vi "Logging Message Loop.vi"(8 "error in (no error)":errorcluster, 9 "Data Notifier":refnum<notifier>, 10 "Data Queue":refnum<queue>, 11 "Message Queues":T1) -> (0 "error out":errorcluster)   [LabVIEW 2022 SP3, in "Logging.lvlib"]
doc: "The message loop subVI to handle messages pertaining to logging data."
uses:
  Logging.lvlib
  support/Message Queue/All Message Queues.ctl
  support/Message Queue/Message Cluster.ctl
  QueuedLoggedData.ctl
  FFT-Data.ctl
  Logging Configuration.ctl
  support/TDMS-Refs.ctl
  Logging State.ctl
  FiniteMeasurement-DAQmx/controls/Hardware Configuration.ctl
  AcquisitionFilter.ctl
  support/Message Queue/Enqueue Message (Single).vi
  <vilib>/Utility/error.llb/Error Cluster From Error Code.vi
  <vilib>/ErrorRing/Error Ring.xnode
  support/Message Queue/Message Queue.lvlib
  Acquisition/Acquisition.lvlib
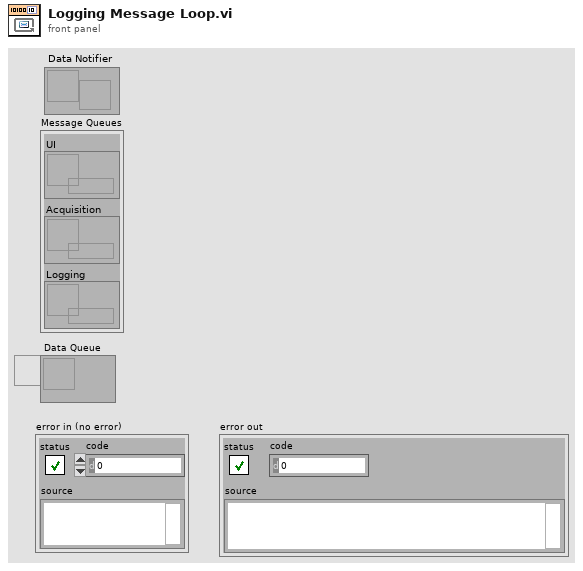
[diagram p1: front panel]
types:
  T1 = typedef "Message Queue.lvlib/All Message Queues.ctl" = cluster{"UI":refnum<queue>, "Acquisition":refnum<queue>, "Logging":refnum<queue>}
  T2 = typedef "Acquisition.lvlib/Hardware Configuration.ctl" = cluster{"Accel-ai0":bool, "Maximum Input":dbl, "Minimum Input":dbl, "Sample Rate":dbl, "Number of Samples":i32, "Accel-ai1":bool, "DAQmx Task":refnum<k21>, "Low Pass Filter":T3}
  T3 = typedef "Acquisition.lvlib/AcquisitionFilter.ctl" = cluster{"Upper Cutoff":dbl, "Lower Cutoff":dbl, "Order":i32}
  T4 = typedef "Logging.lvlib/Logging State.ctl" = cluster{"State":enum16{"Logging", "Not Logging", "Idle"}, "Samples to Save":u32, "Force Trigger":bool, "FFT-Count":i32}
  T5 = typedef "Logging.lvlib/Logging Configuration.ctl" = cluster{"Log File Base Path":path, "Samples to Save":u32, "Acquisition Sample Rate":dbl, "SamplesPerChannel":u32, "FFT - Block Size":u32, "FFT - NumberOfAverages":i32, "Trigger - Time":i32, "Trigger - Threshold":dbl, "Trigger - Channel":u32, "Enable Time Trigger":bool, "Enable Threshold Trigger":bool, "Always Log":bool, "Enable Filter":bool, "FilesRefs":T6, "OutputFileFormat":enum16{"TXT", "TDMS"}, "ActualBlockSize":i32, "HasBeenTriggeredAlready":bool, "Start Time":timestamp}
  T6 = typedef "TDMS-Refs.ctl" = cluster{"TimeDomainTDMSRef":refnum<k34>, "FreuencyDomainTDMSRef":refnum<k34>, "TXT-FileRef":refnum<file>}
  T7 = enum16{"open", "open or create", "create or replace", "create", "open (read-only)"}
  T8 = enum16{"open", "replace", "create", "open or create", "replace or create", "replace or create with confirmation"}
  T9 = typedef "QueuedLoggedData.ctl" = cluster{"RawData":waveform(dbl)[], "FFT ":T10[]}
  T10 = typedef "FFT-Data.ctl" = cluster{"FFT-Mag":cluster{"t0":dbl, "dt":dbl, "Y":dbl[]}, "FFT-Phase":cluster{"t0":dbl, "dt":dbl, "Y":dbl[]}}
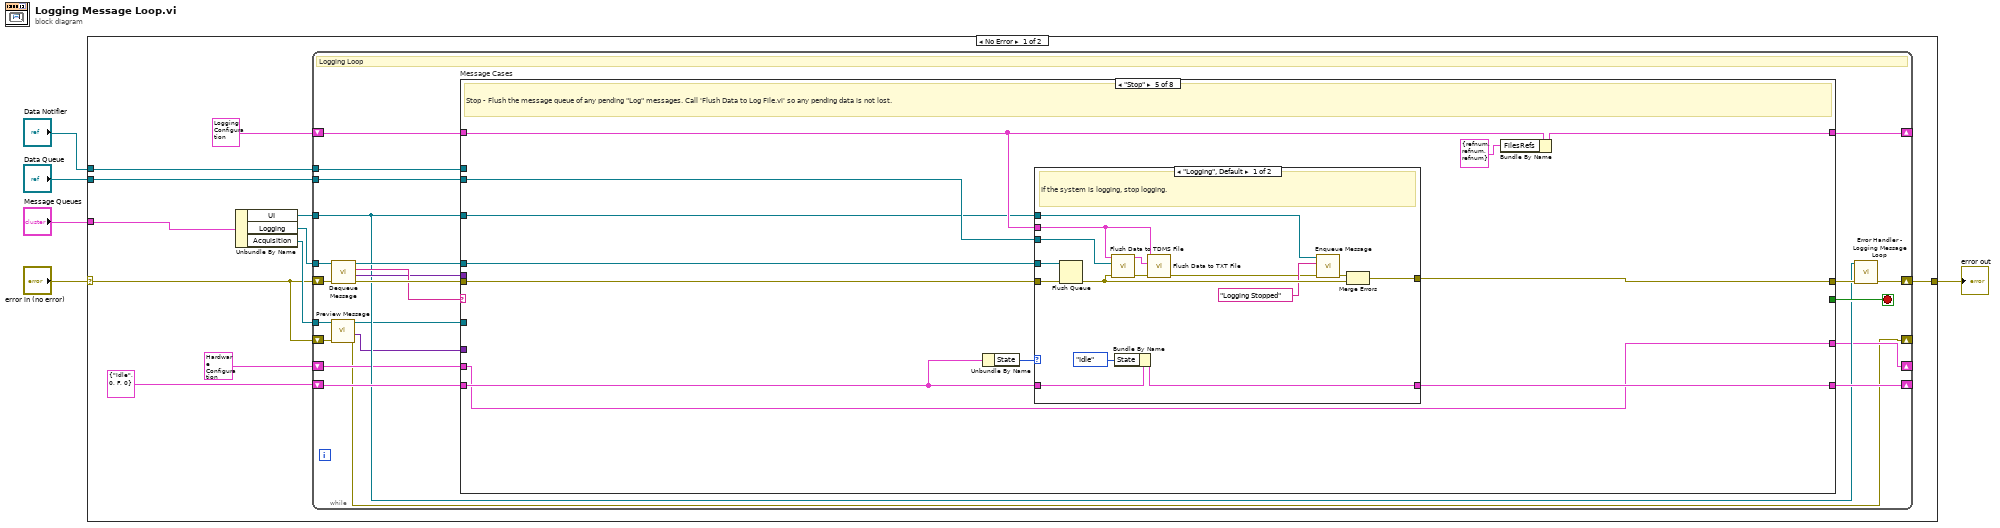
[diagram p0: block diagram]
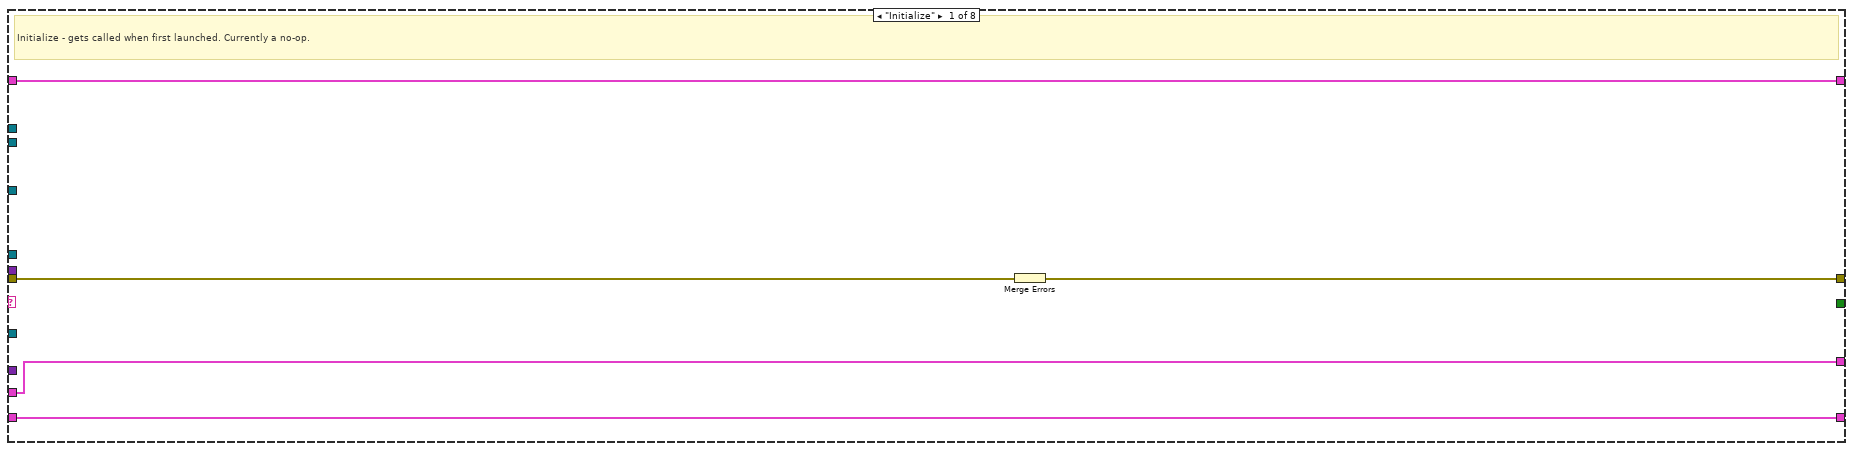
[diagram p2: hidden frame]
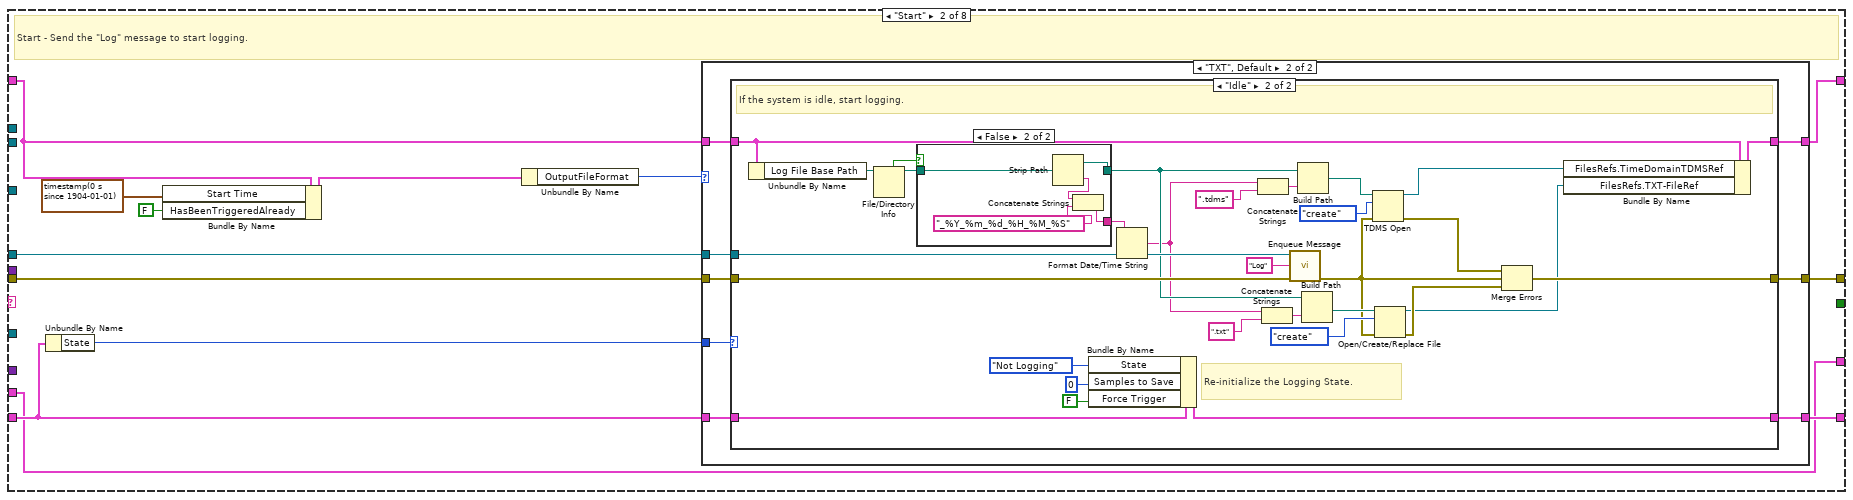
[diagram p3: hidden frame]
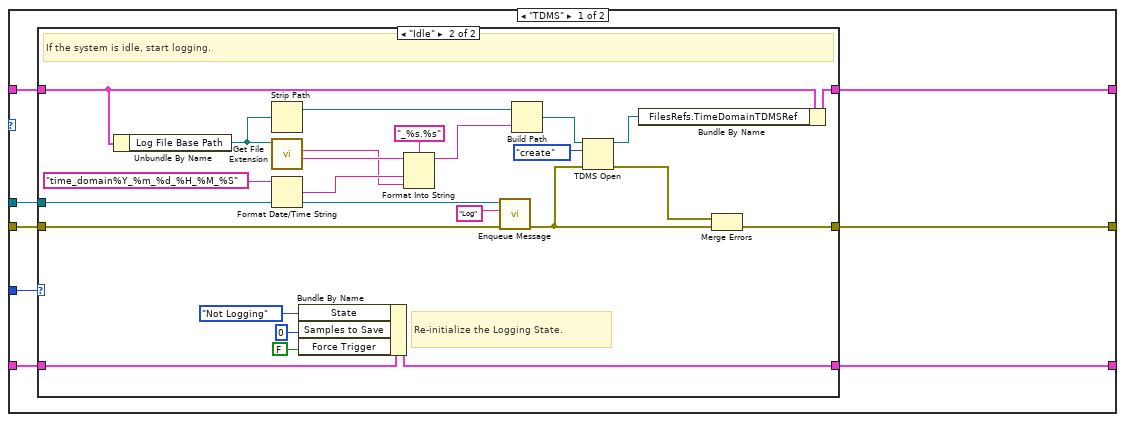
[diagram p4: hidden frame]
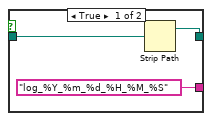
[diagram p7: hidden frame]
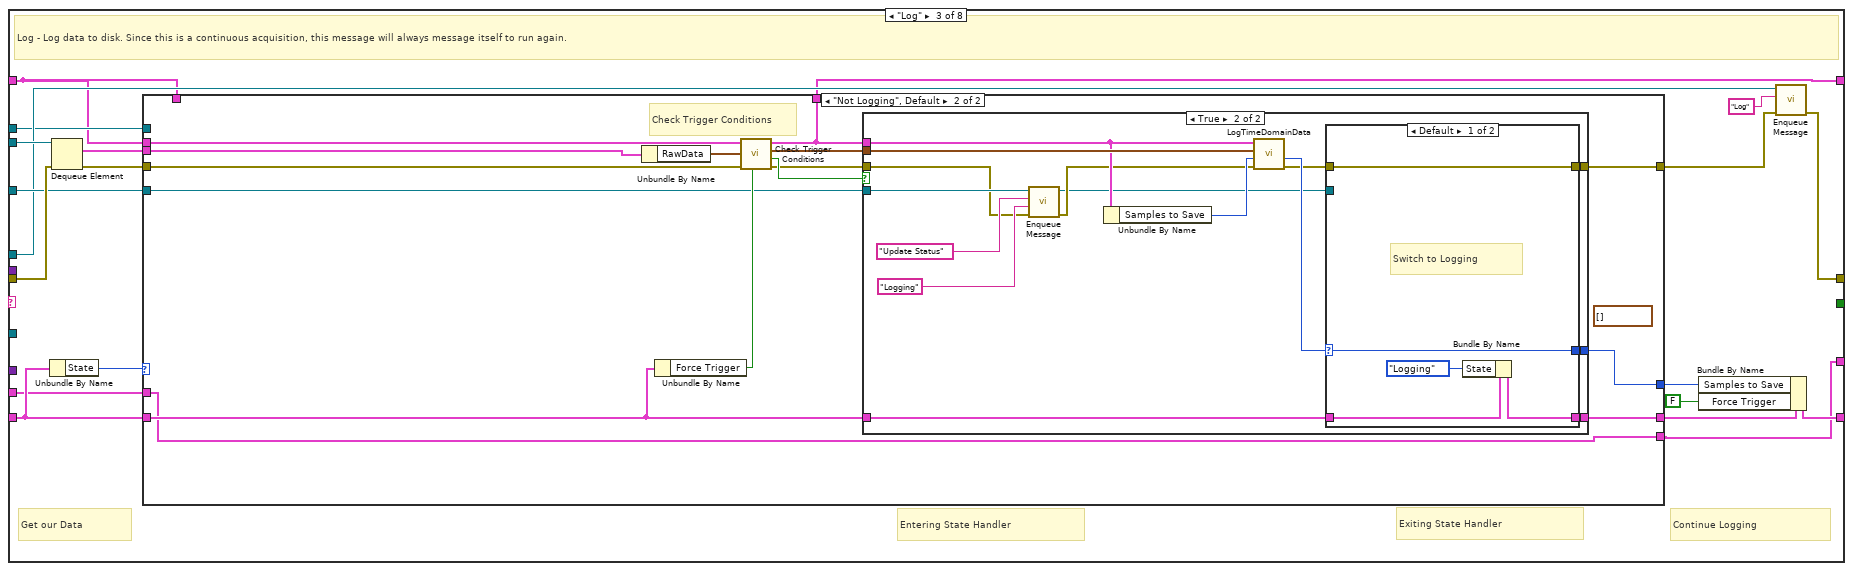
[diagram p8: hidden frame]
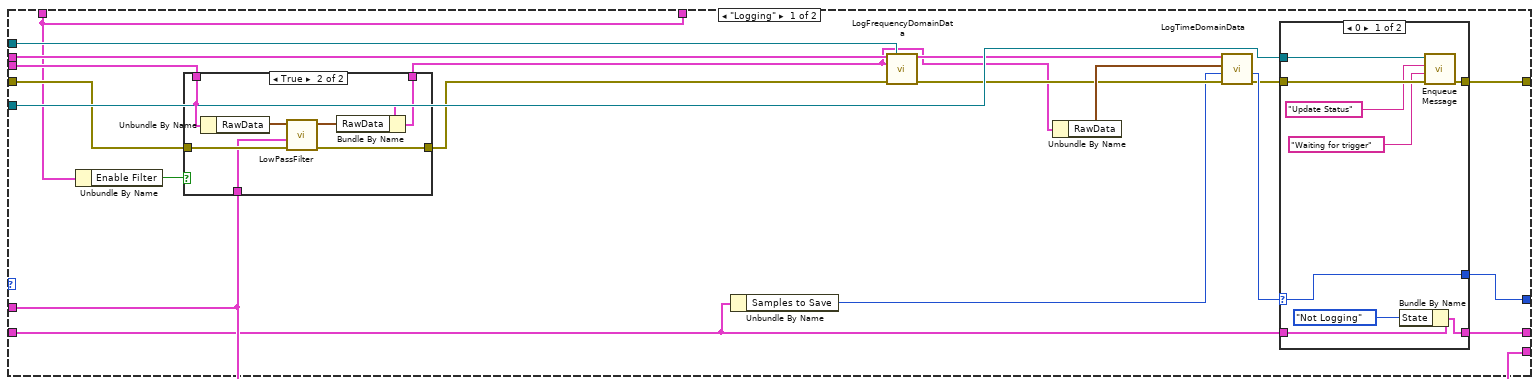
[diagram p9: hidden frame]
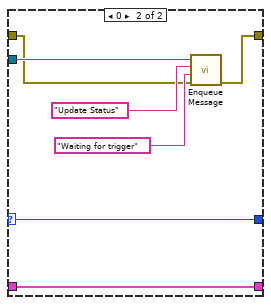
[diagram p13: hidden frame]
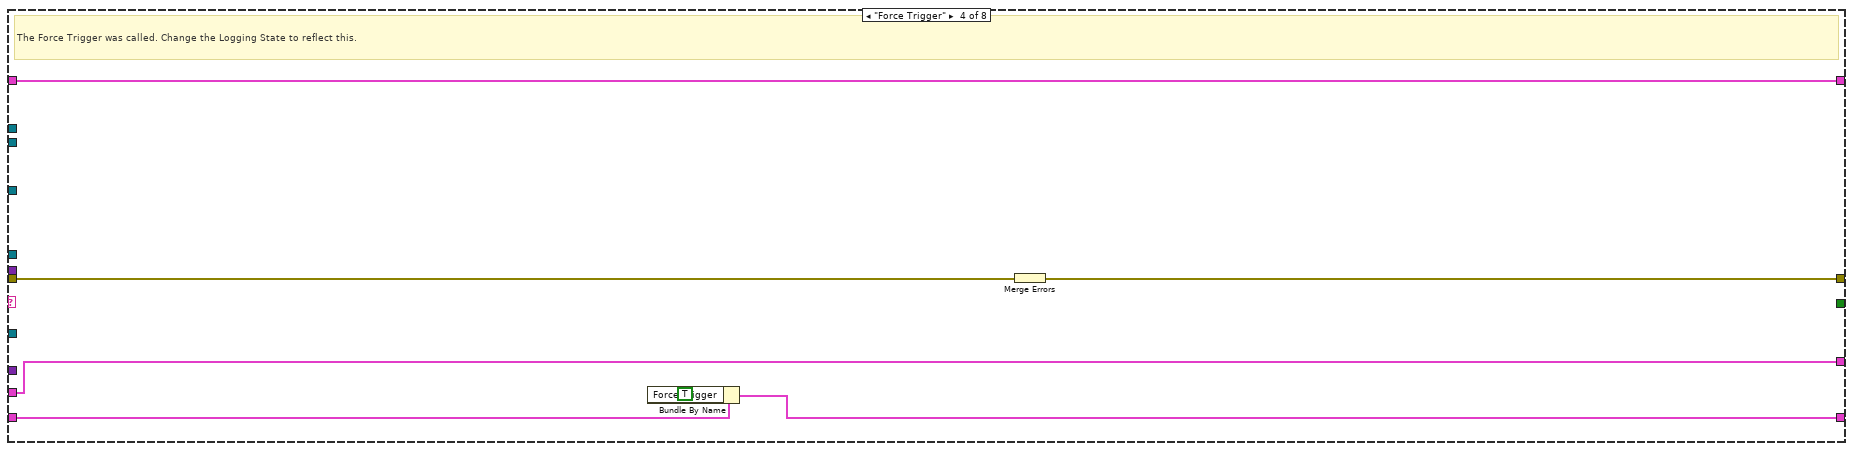
[diagram p14: hidden frame]
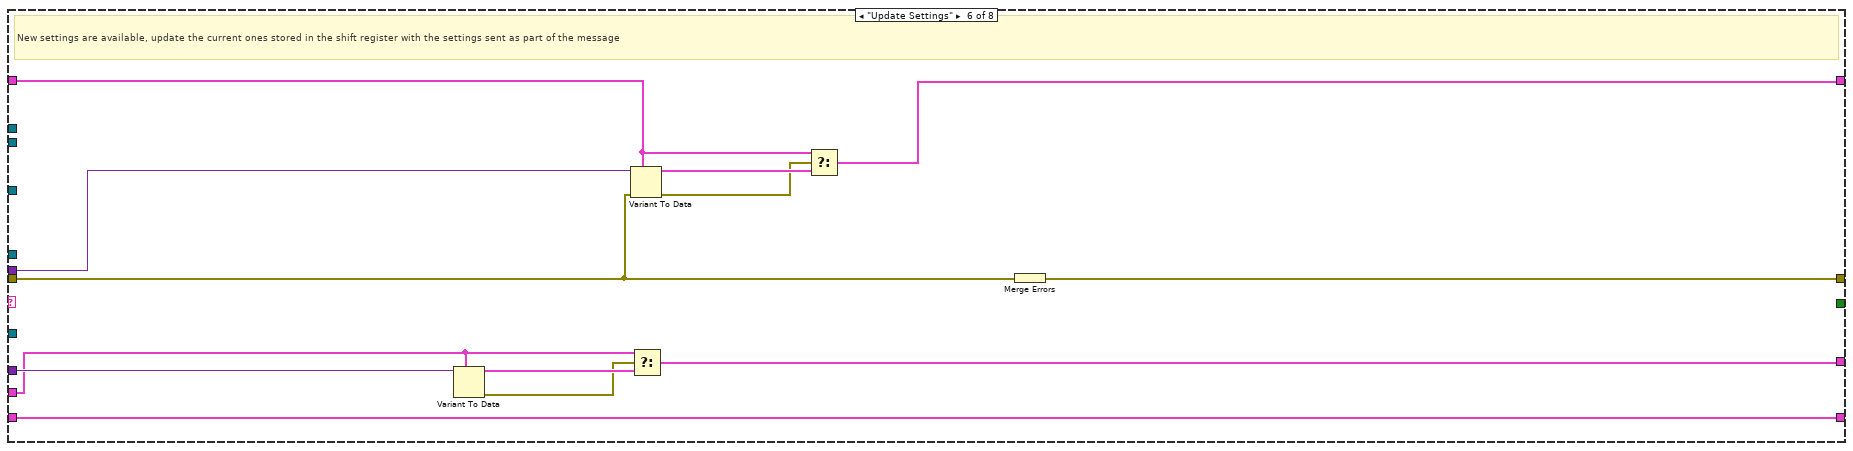
[diagram p16: hidden frame]
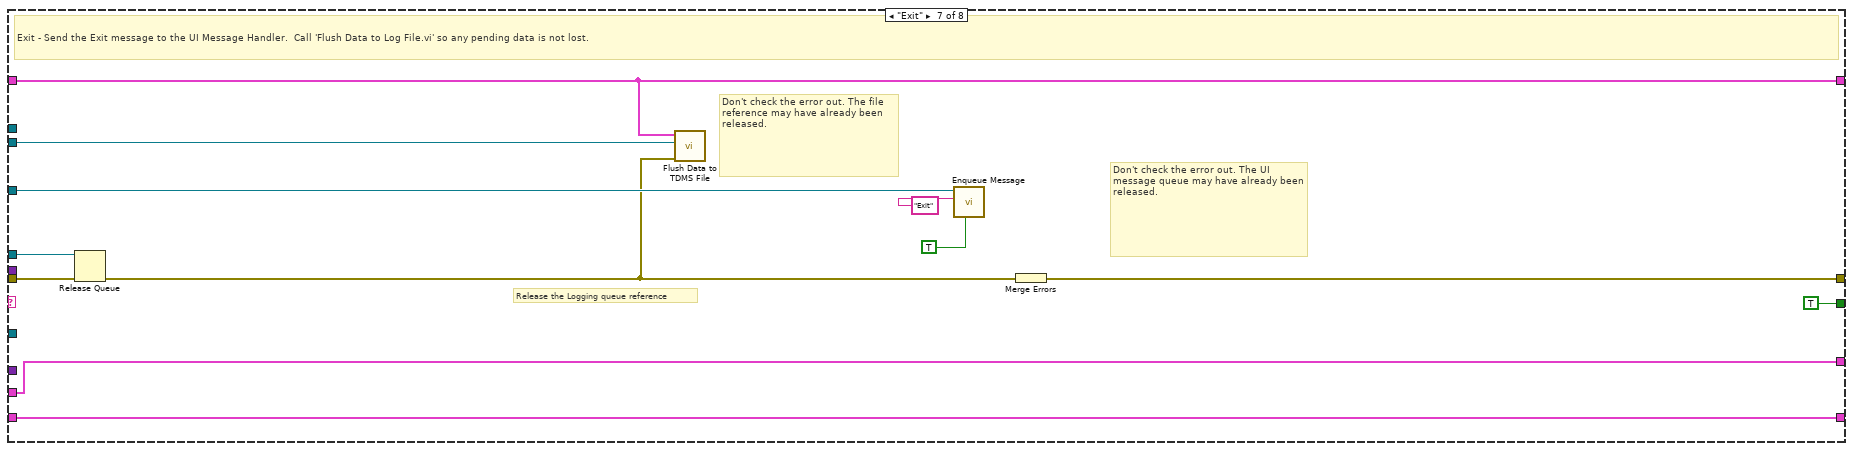
[diagram p17: hidden frame]
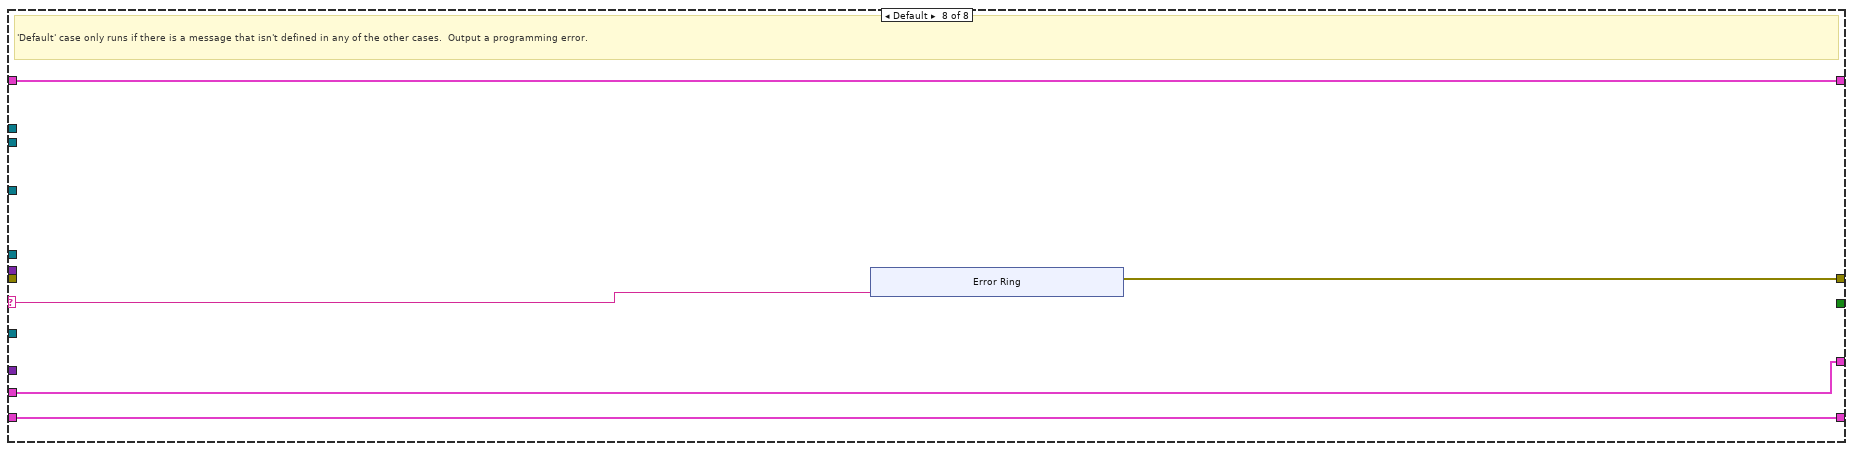
[diagram p18: hidden frame]
diagram:
  n1 = case shown="No Error" "error in (no error)" {
    selector: "error in (no error)" -> [w7 w320]
    tunnel: "Message Queues" -> [w16 _]
    tunnel: [w14 w320] -> w4
    tunnel: "Data Queue" -> [w13 _]
    tunnel: "Data Notifier" -> [w9 _]
    frame No Error {
      n2 = Unbundle By Name(w16) -> ("UI"=w12:refnum<queue>, "Logging"=w15:refnum<queue>, "Acquisition"=w8:refnum<queue>)
      n3 = while {
        tunnel: w15 -> [w31]
        shift-right: [w38] -> _
        shift-left: T5 {"Log File Base Path"=path "", "Samples to Save"=0, "Acquisition Sample Rate"=0.0, "SamplesPerChannel"=0, "FFT - Block Size"=0, "FFT - NumberOfAverages"=0, "Trigger - Time"=0, "Trigger - Threshold"=0.0, "Trigger - Channel"=0, "Enable Time Trigger"=FALSE, "Enable Threshold Trigger"=FALSE, "Always Log"=FALSE, "Enable Filter"=FALSE, "FilesRefs"={"TimeDomainTDMSRef"=refnum, "FreuencyDomainTDMSRef"=refnum, "TXT-FileRef"=refnum}, "OutputFileFormat"=enum."TXT", "ActualBlockSize"=0, "HasBeenTriggeredAlready"=FALSE, "Start Time"=timestamp(0 s since 1904-01-01)} ("Logging Configuration") -> [w39]
        shift-right: [w26] -> w14
        shift-left: w7 -> [w36]
        tunnel: w12 -> [w25]
        tunnel: w13 -> [w30]
        shift-right: [w28] -> _
        shift-left: T4 {"State"=enum."Idle", "Samples to Save"=0, "Force Trigger"=FALSE, "FFT-Count"=0} -> [w29]
        tunnel: w9 -> [w24]
        tunnel: w8 -> [w23]
        shift-right: [w17] -> _
        shift-left: w7 -> [w22]
        shift-right: [w18] -> _
        shift-left: T2 {"Accel-ai0"=FALSE, "Maximum Input"=0.0, "Minimum Input"=0.0, "Sample Rate"=0.0, "Number of Samples"=0, "Accel-ai1"=FALSE, "DAQmx Task"="", "Low Pass Filter"={"Upper Cutoff"=350.0, "Lower Cutoff"=350.0, "Order"=350}} ("Hardware Configuration") -> [w20]
        stop <- w37 stop-if-true
        # "Logging Loop"
        n4 = call "Preview Message.vi"("error in (no error)"=w22, "Message Queue"=w23) -> ("error out"=w17:errorcluster, "Message Data"=w19:variant, "dup Message Queue"=w21:refnum<queue>)  [unwired: 6 in, 1 out]
        n5 = call "Dequeue Message.vi"("error in (no error)"=w36, "Message Queue"=w31) -> ("error out"=w35:errorcluster, "Message Data"=w33:variant, "Message"=w34:string, "dup Message Queue"=w32:refnum<queue>)  [unwired: 6 in]
        n6 = case "Message Cases" shown="\"Stop\"" w34 {
          selector: w34 -> [_ _ _ _ _ _ _ w309]
          tunnel: w32 -> [_ w56 w151 _ w263 _ w301 _]
          tunnel: w35 -> [w42 w55 w160 w253 w264 w289 w304 _]
          tunnel: [w44 w57 w161 w251 w265 w295 w306 w310] -> w27
          tunnel: w39 -> [w43 w50 w142 w252 w261 w293 w300 w312]
          tunnel: [w43 w54 w143 w252 w262 w290 w300 w312] -> w38
          tunnel: [_ _ _ _ _ _ TRUE _] -> w37
          tunnel: w33 -> [_ _ _ _ _ w294 _ _]
          tunnel: w25 -> [_ _ w155 _ w259 _ w305 _]
          tunnel: w30 -> [_ _ w152 _ w260 _ w299 _]
          tunnel: w29 -> [w41 w52 w158 w250 w257 w288 w297 w311]
          tunnel: [w41 w53 w154 w249 w256 w288 w297 w311] -> w28
          tunnel: w24 -> [_ _ w146 _ _ _ _ _]
          tunnel: w21 -> [_ _ _ _ _ _ _ _]
          tunnel: w20 -> [w40 w48 w145 w247 w254 w284 w296 w308]
          tunnel: w19 -> [_ _ _ _ _ w285 _ _]
          tunnel: [w40 w48 w144 w247 w254 w283 w296 w308] -> w18
          frame "Initialize" {
            # "Initialize - gets called when first launched. Currently a no-op."
            n7 = Merge Errors(w42) -> (w44:errorcluster)
          }
          frame "Start" {
            # "Start - Send the \"Log\" message to start logging."
            n8 = Unbundle By Name(w52) -> ("State"=w51:enum16{"Logging", "Not Logging", "Idle"})
            n9 = Bundle By Name(cluster=w50, "Start Time"=timestamp(0 s since 1904-01-01), "HasBeenTriggeredAlready"=FALSE) -> (w47:T5)
            n10 = Unbundle By Name(w47) -> ("OutputFileFormat"=w49:enum16{"TXT", "TDMS"})
            n11 = case shown="\"TXT\", Default" w49 {
              tunnel: [w65 w100] -> w57
              tunnel: w56 -> [w64 w99]
              tunnel: w55 -> [w63 w98]
              tunnel: [w62 w97] -> w54
              tunnel: [w61 w96] -> w53
              tunnel: w52 -> [w60 w95]
              tunnel: w51 -> [w59 w94]
              tunnel: w50 -> [w58 w93]
              frame "TDMS" {
                n12 = case shown="\"Idle\"" w59 {
                  tunnel: [w67 w92] -> w65
                  tunnel: w64 -> [_ w91]
                  tunnel: w63 -> [w67 w89]
                  tunnel: w58 -> [w68 w80]
                  tunnel: [w68 w77] -> w62
                  tunnel: w60 -> [w66 w73]
                  tunnel: [w66 w72] -> w61
                  frame "Logging", Default {
                    # "The system is already running. Ignore the \"Start\" message."
                  }
                  frame "Idle" {
                    # "Re-initialize the Logging State."
                    # "If the system is idle, start logging."
                    n13 = Unbundle By Name(w80) -> ("Log File Base Path"=w87:path)
                    n14 = Strip Path(path=w87) -> (stripped path=w86:path)  [unwired: 1 out]
                    n15 = call <vilib>:"Get File Extension.vi"("file"=w87) -> ("filename without extension"=w85:string, "lowercase file extension"=w82:string)  [unwired: 6 in, 3 out]
                    n16 = Format Date/Time String(time format string (%c)="time_domain%Y_%m_%d_%H_%M_%S") -> (date/time string=w83:string)  [unwired: 2 in]
                    n17 = Bundle By Name(cluster=w73, "State"=enum16{"Logging", "Not Logging"}."Not Logging", "Samples to Save"=u32 0 ("Reads to Save"), "Force Trigger"=FALSE) -> (w72:T4)
                    n18 = Format Into String(format string="_%s.%s", initial string=w85, w83, w82) -> (resulting string=w81:string)  [unwired: 1 in, 1 out]
                    n19 = call-poly "Enqueue Message.vi"("error in (no error)"=w89, "Message"="Log", "Message Queue"=w91) -> ("error out"=w75:errorcluster)  [unwired: 7 in, 1 out]
                    n20 = Build Path(base path=w86, name or relative path=w81) -> (appended path=w78:path)
                    n21 = TDMS Open(8:w75, 10:T7."create" ("operation (0:open)"), 11:w78) -> (0:w74:errorcluster, 3:w79:refnum<k34>)  [unwired: 4 in]
                    n22 = Bundle By Name(cluster=w80, "FilesRefs.TimeDomainTDMSRef"=w79) -> (w77:T5)
                    n23 = Merge Errors(w74, w75) -> (w92:errorcluster)
                  }
                }
              }
              frame "TXT", Default {
                n24 = case shown="\"Idle\"" w94 {
                  tunnel: [w102 w133] -> w100
                  tunnel: w99 -> [_ w132]
                  tunnel: w98 -> [w102 w130]
                  tunnel: w93 -> [w103 w128]
                  tunnel: [w103 w125] -> w97
                  tunnel: w95 -> [w101 w122]
                  tunnel: [w101 w121] -> w96
                  frame "Logging", Default {
                    # "The system is already running. Ignore the \"Start\" message."
                  }
                  frame "Idle" {
                    # "Re-initialize the Logging State."
                    # "If the system is idle, start logging."
                    n25 = Unbundle By Name(w128) -> ("Log File Base Path"=w117:path)
                    n26 = File/Directory Info(path=w117) -> (path out=w105:path, directory=w104:bool)  [unwired: 1 in, 5 out]
                    n27 = case shown="False" w104 {
                      tunnel: ["log_%Y_%m_%d_%H_%M_%S" ("time format string (%c)") w137] -> w129
                      tunnel: [w135 w141] -> w107
                      tunnel: w105 -> [w134 w140]
                      frame True {
                        n28 = Strip Path(path=w134) -> (stripped path=w135:path)  [unwired: 1 out]
                      }
                      frame False {
                        n29 = Strip Path(path=w140) -> (stripped path=w141:path, name=w139:string)
                        n30 = Concatenate Strings(w139, "_%Y_%m_%d_%H_%M_%S" ("time format string (%c)")) -> (w137:string)
                      }
                    }
                    n31 = Bundle By Name(cluster=w122, "State"=enum16{"Logging", "Not Logging"}."Not Logging", "Samples to Save"=u32 0 ("Reads to Save"), "Force Trigger"=FALSE) -> (w121:T4)
                    n32 = Format Date/Time String(time format string (%c)=w129) -> (date/time string=w106:string)  [unwired: 2 in]
                    n33 = Concatenate Strings(w106, ".tdms" ("input 2")) -> (w116:string)
                    n34 = Concatenate Strings(w106, ".txt" ("input 2")) -> (w114:string)
                    n35 = call-poly "Enqueue Message.vi"("error in (no error)"=w130, "Message"="Log", "Message Queue"=w132) -> ("error out"=w110:errorcluster)  [unwired: 7 in, 1 out]
                    n36 = Build Path(base path=w107, name or relative path=w116) -> (appended path=w126:path)
                    n37 = Build Path(base path=w107, name or relative path=w114) -> (appended path=w112:path)
                    n38 = TDMS Open(8:w110, 10:T7."create" ("operation (0:open)"), 11:w126) -> (0:w123:errorcluster, 3:w127:refnum<k34>)  [unwired: 4 in]
                    n39 = Open/Create/Replace File(file path (use dialog)=w112, error in=w110, operation (0:open)=T8."create") -> (refnum out=w108:refnum<file>, error out=w109:errorcluster)  [unwired: 3 in, 1 out]
                    n40 = Merge Errors(w123, w110, w109) -> (w133:errorcluster)
                    n41 = Bundle By Name(cluster=w128, "FilesRefs.TimeDomainTDMSRef"=w127, "FilesRefs.TXT-FileRef"=w108) -> (w125:T5)
                  }
                }
              }
            }
          }
          frame "Log" {
            # "Exiting State Handler"
            # "Continue Logging"
            # "Entering State Handler"
            # "Get our Data"
            # "Log - Log data to disk. Since this is a continuous acquisition, this message will always message itself to run again."
            n42 = Unbundle By Name(w158) -> ("State"=w159:enum16{"Logging", "Not Logging", "Idle"})
            n43 = Dequeue Element(queue=w152, error in (no error)=w160) -> (element=w157:T9, error out=w156:errorcluster)  [unwired: 1 in, 2 out]
            n44 = case shown="\"Not Logging\", Default" w159 {
              tunnel: [w180 w210] -> w150
              tunnel: w158 -> [w163 w208]
              tunnel: w157 -> [w166 w216]
              tunnel: w156 -> [w169 w215]
              tunnel: w142 -> [w172 w217]
              tunnel: w155 -> [w176 w207]
              tunnel: [w177 w209] -> w149
              tunnel: [w179 w206] -> w148
              tunnel: w146 -> [w170 _]
              tunnel: w142 -> [w162 _]
              tunnel: w145 -> [w164 w204]
              tunnel: [w164 w204] -> w144
              tunnel: [w162 w203] -> w143
              frame "Logging" {
                n45 = Unbundle By Name(w162) -> ("Enable Filter"=w165:bool)
                n46 = case shown="True" w165 {
                  tunnel: w169 -> [w183 w189]
                  tunnel: [w183 w188] -> w168
                  tunnel: [w182 w186] -> w167
                  tunnel: w166 -> [w182 w185]
                  tunnel: w164 -> [_ w184]
                  frame False {
                  }
                  frame True {
                    n47 = Unbundle By Name(w185) -> ("RawData"=w190:waveform(dbl)[])
                    n48 = call "LowPassFilter.vi"("error in (no error)"=w189, "Àcquiring Configurations"=w184, "InputData"=w190) -> ("error out"=w188:errorcluster, "OutputData"=w187:waveform(dbl)[])  [unwired: 7 in]
                    n49 = Bundle By Name(cluster=w185, "RawData"=w187) -> (w186:T9)
                  }
                }
                n50 = Unbundle By Name(w163) -> ("Samples to Save"=w171:u32)
                n51 = call "LogFrequencyDomainData.vi"("Logging Configuration Input"=w172, "Data Notifier"=w170, "QueuedDataInput"=w167, "error in (no error)"=w168) -> ("Logging Configuration Output"=w173:T5, "error out"=w174:errorcluster)  [unwired: 10 in]
                n52 = Unbundle By Name(w167) -> ("RawData"=w175:waveform(dbl)[])
                n53 = call "LogTimeDomainData.vi"("error in (no error)"=w174, "Samples to Save In"=w171, "Data"=w175, "Logging Configuration"=w173) -> ("error out"=w178:errorcluster, "Samples to Save Out"=w181:u32)  [unwired: 6 in]
                n54 = case shown="0" w181 {
                  selector: w181 -> [w196 w202]
                  tunnel: w178 -> [w194 w201]
                  tunnel: [w195 w201] -> w177
                  tunnel: w163 -> [w198 w200]
                  tunnel: [w197 w200] -> w180
                  tunnel: [w196 w202] -> w179
                  tunnel: w176 -> [w191 _]
                  frame 0 {
                    n55 = Bundle By Name(cluster=w198, "State"=enum16{"Logging", "Not Logging"}."Not Logging") -> (w197:T4)
                    n56 = call-poly "Enqueue Message.vi"("error in (no error)"=w194, "Message Data"="Waiting for trigger" ("Waiting for trigger"), "Message"="Update Status", "Message Queue"=w191) -> ("error out"=w195:errorcluster)  [unwired: 6 in, 1 out]
                  }
                  frame Default {
                    # "Continue in our same State."
                  }
                }
              }
              frame "Not Logging", Default {
                (unwired) waveform(dbl)[] []
                # "Check Trigger Conditions"
                n57 = Unbundle By Name(w216) -> ("RawData"=w205:waveform(dbl)[])
                n58 = Unbundle By Name(w208) -> ("Force Trigger"=w214:bool)
                n59 = call "Check Trigger Conditions.vi"("Force Trigger?"=w214, "error in (no error)"=w215, "Waveform Data In"=w205, "Logging Configuration In"=w217) -> ("error out"=w212:errorcluster, "Trigger Conditions Met?"=w213:bool, "Waveform Data Out (copy)"=w211:waveform(dbl)[], "Logging Configuration Out"=w203:T5)  [unwired: 4 in]
                n60 = case shown="True" w213 {
                  tunnel: w212 -> [w218 w228]
                  tunnel: w211 -> [_ w234]
                  tunnel: w203 -> [_ w233]
                  tunnel: w208 -> [w219 w224]
                  tunnel: [w219 w223] -> w210
                  tunnel: [w218 w221] -> w209
                  tunnel: w207 -> [_ w232]
                  tunnel: [_ w225] -> w206
                  frame False {
                  }
                  frame True {
                    n61 = call-poly "Enqueue Message.vi"("error in (no error)"=w228, "Message Data"="Logging" ("Logging"), "Message"="Update Status", "Message Queue"=w232) -> ("error out"=w227:errorcluster, "dup Message Queue"=w220:refnum<queue>)  [unwired: 6 in]
                    n62 = Unbundle By Name(w233) -> ("Samples to Save"=w229:u32)
                    n63 = call "LogTimeDomainData.vi"("error in (no error)"=w227, "Samples to Save In"=w229, "Data"=w234, "Logging Configuration"=w233) -> ("error out"=w222:errorcluster, "Samples to Save Out"=w226:u32)  [unwired: 6 in]
                    n64 = case shown="Default" w226 {
                      selector: w226 -> [w239 w246]
                      tunnel: [w239 w246] -> w225
                      tunnel: [w236 w245] -> w223
                      tunnel: w224 -> [w237 w245]
                      tunnel: w222 -> [w235 w241]
                      tunnel: [w235 w240] -> w221
                      tunnel: w220 -> [_ w244]
                      frame Default {
                        # "Switch to Logging"
                        n65 = Bundle By Name(cluster=w237, "State"=enum16{"Logging", "Not Logging"}."Logging") -> (w236:T4)
                      }
                      frame 0 {
                        n66 = call-poly "Enqueue Message.vi"("error in (no error)"=w241, "Message Data"="Waiting for trigger" ("Waiting for trigger"), "Message"="Update Status", "Message Queue"=w244) -> ("error out"=w240:errorcluster)  [unwired: 6 in, 1 out]
                      }
                    }
                  }
                }
              }
            }
            n67 = Bundle By Name(cluster=w150, "Samples to Save"=w148, "Force Trigger"=FALSE) -> (w154:T4)
            n68 = call-poly "Enqueue Message.vi"("error in (no error)"=w149, "Message"="Log", "Message Queue"=w151) -> ("error out"=w161:errorcluster)  [unwired: 7 in, 1 out]
          }
          frame "Force Trigger" {
            # "The Force Trigger was called. Change the Logging State to reflect this."
            n69 = Bundle By Name(cluster=w250, "Force Trigger"=TRUE) -> (w249:T4)
            n70 = Merge Errors(w253) -> (w251:errorcluster)
          }
          frame "Stop" {
            # "Stop - Flush the message queue of any pending \"Log\" messages. Call 'Flush Data to Log File.vi' so any pending data is not lost."
            n71 = Unbundle By Name(w257) -> ("State"=w258:enum16{"Logging", "Not Logging", "Idle"})
            n72 = case shown="\"Logging\", Default" w258 {
              tunnel: [w280 w282] -> w265
              tunnel: w264 -> [w279 w282]
              tunnel: w263 -> [w278 _]
              tunnel: w261 -> [w266 _]
              tunnel: w260 -> [w277 _]
              tunnel: w259 -> [w273 _]
              tunnel: w257 -> [w271 w281]
              tunnel: [w270 w281] -> w256
              frame "Logging", Default {
                # "If the system is logging, stop logging."
                n73 = Flush Queue(queue=w278, error in (no error)=w279) -> (error out=w276:errorcluster)  [unwired: 2 out]
                n74 = call "Flush Data to TDMS File.vi"("error in (no error)"=w276, "Data Queue"=w277, "Logging Configuration"=w266) -> ("error out"=w275:errorcluster, "remaining elements"=w267:T9[])  [unwired: 7 in]
                n75 = Bundle By Name(cluster=w271, "State"=enum16{"Logging", "Not Logging", "Idle"}."Idle") -> (w270:T4)
                n76 = call "Flush Data to TXT File.vi"("error in (no error)"=w275, "remaining elements"=w267, "Logging Configuration Input"=w266) -> ("error out"=w268:errorcluster)  [unwired: 8 in]
                n77 = call-poly "Enqueue Message.vi"("error in (no error)"=w268, "Message"="Logging Stopped", "Message Queue"=w273) -> ("error out"=w274:errorcluster)  [unwired: 7 in, 1 out]
                n78 = Merge Errors(w274, w276) -> (w280:errorcluster)
              }
              frame "Idle" {
                # "The system is already idle. Ignore the \"Stop\" message."
              }
            }
            n79 = Bundle By Name(cluster=w261, "FilesRefs"=T6 {"TimeDomainTDMSRef"=refnum, "FreuencyDomainTDMSRef"=refnum, "TXT-FileRef"=refnum}) -> (w262:T5)
          }
          frame "Update Settings" {
            # "New settings are available, update the current ones stored in the shift register with the settings sent as part of the message"
            n80 = Variant To Data(type=w284, Variant=w285) -> (data=w287:T2, error out=w286:errorcluster)  [unwired: 1 in]
            n81 = Variant To Data(error in=w289, type=w293, Variant=w294) -> (data=w292:T5, error out=w291:errorcluster)
            n82 = Select(t=w284, s=w286, f=w287) -> (s? t:f=w283:T2)
            n83 = Select(t=w293, s=w291, f=w292) -> (s? t:f=w290:T5)
            n84 = Merge Errors(w289) -> (w295:errorcluster)
          }
          frame "Exit" {
            # "Don't check the error out. The file reference may have already been released."
            # "Release the Logging queue reference"
            # "Don't check the error out. The UI message queue may have already been released."
            # "Exit - Send the Exit message to the UI Message Handler.  Call 'Flush Data to Log File.vi' so any pending data is not lost."
            n85 = Release Queue(queue=w301, error in (no error)=w304) -> (error out=w298:errorcluster)  [unwired: 1 in, 2 out]
            n86 = call "Flush Data to TDMS File.vi"("error in (no error)"=w298, "Data Queue"=w299, "Logging Configuration"=w300) -> ()  [unwired: 7 in, 2 out]
            n87 = call-poly "Enqueue Message.vi"("Priority Message? (F)"=TRUE, "Message"="Exit", "Message Queue"=w305) -> ()  [unwired: 7 in, 2 out]
            n88 = Merge Errors(w298) -> (w306:errorcluster)
          }
          frame Default {
            # "'Default' case only runs if there is a message that isn't defined in any of the other cases.  Output a programming error."
            n89 = xnode "Error Ring"("parameter 0"=w309) -> ("error out"=w310:errorcluster)
          }
        }
        n90 = call "Error Handler - Logging Message Loop.vi"("error in (no error)"=w27, "Message Queue"=w25) -> ("dup error in"=w26:errorcluster)  [unwired: 8 in, 1 out]
      }
    }
    frame Error {
    }
  }
  "error out" <- w4
